vi "TestFFTOrder.vi"(8 "振动判定":T1, 9 "振动判定范围":T2, 10 "spectrum info":T3[](array[typedef]) {"x-axis units" items=["Time (s)"=0, "Frequency-CB (Hz)"=1, "Frequency-CPB (Hz)"=1248, "Frequency-Arbitrary (Hz)"=2357, "Quefrency (s)"=2, "Revolutions (rev)"=3, "Order"=4, "Speed (RPM)"=11, "Speed (rad/s)"=21, "Index"=65535]; "weighting filter" items=["Linear", "A-weighting", "B-weighting", "C-weighting", "ITU-R 468-4", "Dolby", "CCITT", "C-message", "Wb", "Wc", "Wd", "We", "Wf", "Wh", "Wj", "Wk", "Wm", "AES17 20 kHz lowpass", "AES17 40 kHz lowpass", "AES17 20 kHz highpass", "AES17 40 kHz highpass"]; "dB reference [EU]" format="%.2f"; "engineering units" items=["custom..."=0, "V"=1, "A"=21, "C"=30, "pC"=31, "s"=32, "-"=29, "Pa"=2, "N"=20, "g"=3, "m/s^2"=4, "m/s"=5, "m"=6, "mm/s"=12, "mm"=13, "micron/s"=14, "micron"=15, "in/s^2"=7, "in/s"=8, "in"=9, "mil/s"=10, "mil"=11, "rad/s^2"=16, "rad/s"=17, "rad"=18, "deg/s^2"=26, "deg/s"=27, "deg"=28, "RPM"=22, "cycle/s^2"=23, "Hz"=24, "cycle"=25, "strain"=19]; "spectral info"."window" items=["None "=0, "Hanning"=1, "Hamming"=2, "Blackman-Harris"=3, "Exact Blackman"=4, "Blackman"=5, "Flat Top"=6, "4 Term B-Harris "=7, "7 Term B-Harris"=8, "Low Sidelobe"=9, "Force - Exponential"=10, "Gaussian"=62]}, 11 "FFT 5":cluster{"x0":dbl, "dx":dbl, "Y":dbl[]}[](graph) caption="spectrum") -> (0 "Limit Specifications":cluster{"x0":dbl, "dx":dbl, "Y":dbl[]}[][](array[cluster]), 1 "数组":cluster{"freq.":dbl, "dB":dbl}[][](array[cluster]), 2 "Test Result":bool[][](array[boolean]), 3 "FFT 2":cluster{"x0":dbl, "dx":dbl, "Y":dbl[]}[](graph))   [LabVIEW 2020]
uses:
  <vilib>/measure/NI_MAPro.lvlib
  <vilib>/measure/mamon.llb/Create Continuous Mask.vi
  <vilib>/addons/_NISVFA/_Spectrum Processing/SVFA Get Spectrum Subset (1 Ch).vi
  <vilib>/addons/_NISVFA/_Spectrum Processing/SVFA Spectrum Peak Search (1 Ch).vi
  <vilib>/measure/mamon.llb/Limit Testing Frequency.vi
  <vilib>/addons/_NISVFA/_Shared subVIs/Controls/svc_Spectrum Type.ctl
  <vilib>/addons/_NISVFA/_Shared subVIs/Controls/svc_Engineering Units Text Ring.ctl
  <vilib>/addons/_NISVFA/_Shared subVIs/Controls/svc_Weighting Filter Text Ring.ctl
  <vilib>/addons/_NISVFA/_Shared subVIs/Controls/svc_X-Axis Units.ctl
  <vilib>/addons/_NISVFA/_Shared subVIs/Controls/svc_Complimentary Spectrum Units.ctl
  <vilib>/addons/_NISVFA/_Shared subVIs/Controls/svc_Spectrum Info.ctl
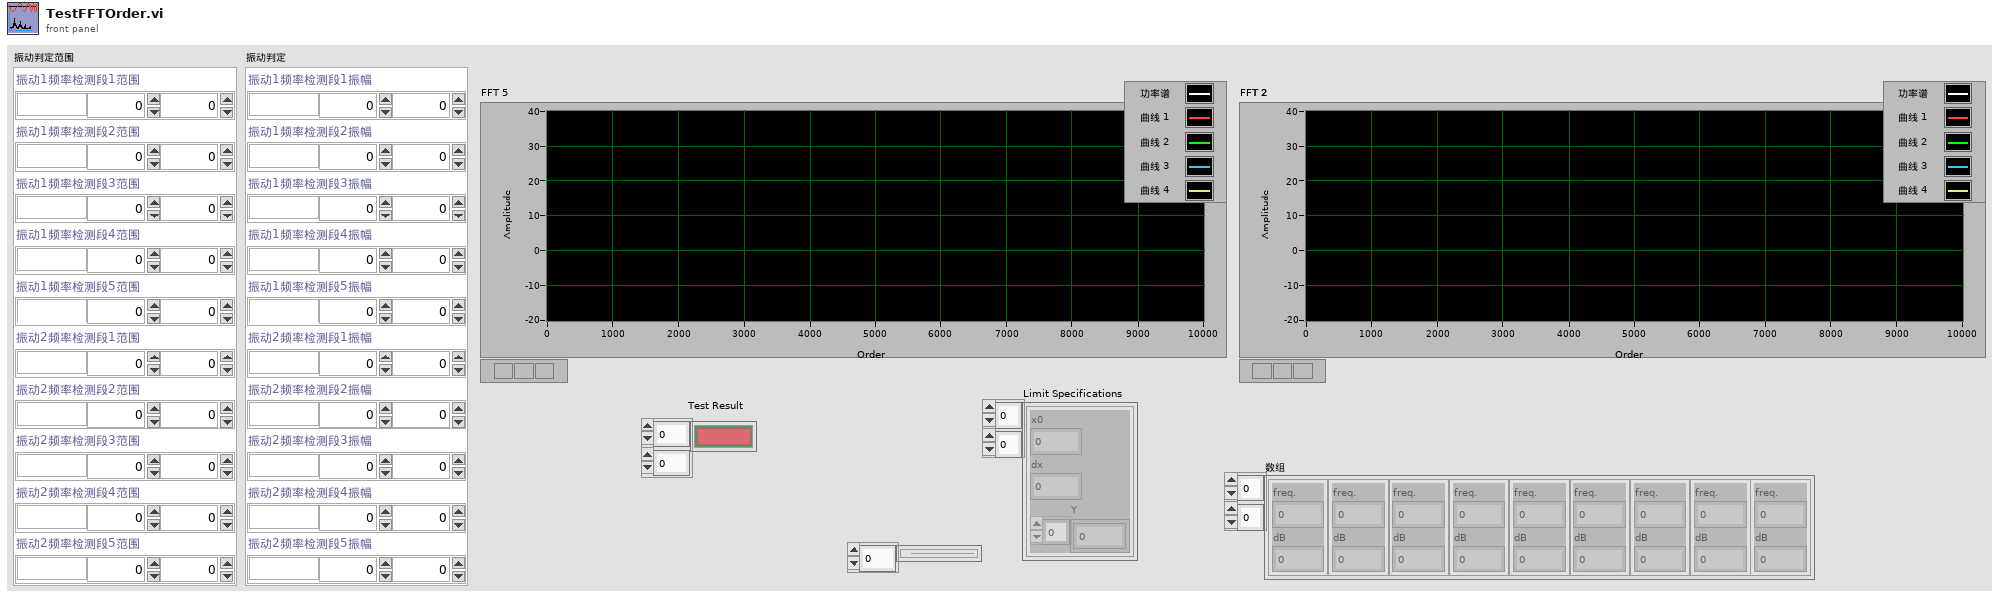
[diagram p1: front panel]
types:
  T1 = cluster{"振动1频率检测段1振幅":cluster{"单位":string, "下限":dbl, "上限":dbl}, "振动1频率检测段2振幅":cluster{"单位":string, "下限":dbl, "上限":dbl}, "振动1频率检测段3振幅":cluster{"单位":string, "下限":dbl, "上限":dbl}, "振动1频率检测段4振幅":cluster{"单位":string, "下限":dbl, "上限":dbl}, "振动1频率检测段5振幅":cluster{"单位":string, "下限":dbl, "上限":dbl}, "振动2频率检测段1振幅":cluster{"单位":string, "下限":dbl, "上限":dbl}, "振动2频率检测段2振幅":cluster{"单位":string, "下限":dbl, "上限":dbl}, "振动2频率检测段3振幅":cluster{"单位":string, "下限":dbl, "上限":dbl}, "振动2频率检测段4振幅":cluster{"单位":string, "下限":dbl, "上限":dbl}, "振动2频率检测段5振幅":cluster{"单位":string, "下限":dbl, "上限":dbl}}
  T2 = cluster{"振动1频率检测段1范围":cluster{"单位":string, "下限":dbl, "上限":dbl}, "振动1频率检测段2范围":cluster{"单位":string, "下限":dbl, "上限":dbl}, "振动1频率检测段3范围":cluster{"单位":string, "下限":dbl, "上限":dbl}, "振动1频率检测段4范围":cluster{"单位":string, "下限":dbl, "上限":dbl}, "振动1频率检测段5范围":cluster{"单位":string, "下限":dbl, "上限":dbl}, "振动2频率检测段1范围":cluster{"单位":string, "下限":dbl, "上限":dbl}, "振动2频率检测段2范围":cluster{"单位":string, "下限":dbl, "上限":dbl}, "振动2频率检测段3范围":cluster{"单位":string, "下限":dbl, "上限":dbl}, "振动2频率检测段4范围":cluster{"单位":string, "下限":dbl, "上限":dbl}, "振动2频率检测段5范围":cluster{"单位":string, "下限":dbl, "上限":dbl}}
  T3 = typedef "svc_Spectrum Info.ctl" = cluster{"channel name":string, "description":string, "x-axis units":T4, "spectral info":cluster{"spectrum type":T5, "linear/dB":enum16{"linear", "dB"}, "window":u16, "window size":i32, "FFT size":i32}, "engineering units":T6, "custom label":string, "dB reference [EU]":dbl, "peak units":enum16{"rms", "peak", "peak-peak"}, "weighting filter":T7, "spectral density?":bool, "unit label":string, "spectrum skewed?":bool, "complimentary spectrum units":T8}
  T4 = typedef "svc_X-Axis Units.ctl" = u16
  T5 = typedef "svc_Spectrum Type.ctl" = enum16{"FFT Spectrum [complex]", "Amplitude [Magnitude]", "Power [Magnitude^2]", "Cross Spectrum [complex]", "Frequency Response [Complex]"}
  T6 = typedef "svc_Engineering Units Text Ring.ctl" = u16
  T7 = typedef "svc_Weighting Filter Text Ring.ctl" = u16
  T8 = typedef "svc_Complimentary Spectrum Units.ctl" = enum16{"none", "radians", "degrees", "cycles", "imaginary"}
  T9 = cluster{"single/multiple":enum16{"Multiple Peaks", "Single Max Peak"}, "threshold":dbl}
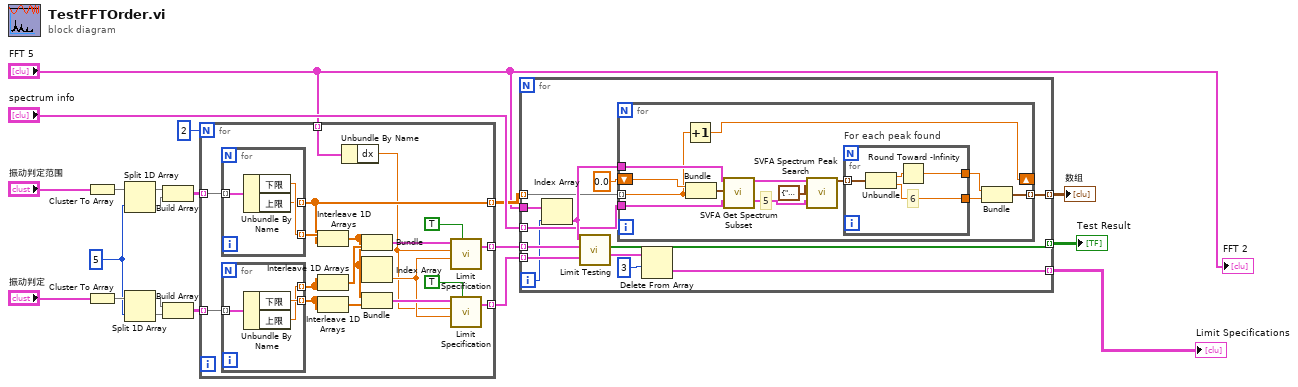
[diagram p0: block diagram]
diagram:
  w16 = 5 ("索引")
  n1 = Cluster To Array(cluster="振动判定范围") -> (array=w18:cluster{"单位":string, "下限":dbl, "上限":dbl}[])
  n2 = Cluster To Array(cluster="振动判定") -> (array=w17:cluster{"单位":string, "下限":dbl, "上限":dbl}[])
  n3 = Split 1D Array(array=w18, index=w16) -> (first subarray=w15:cluster{"单位":string, "下限":dbl, "上限":dbl}[], second subarray=w14:cluster{"单位":string, "下限":dbl, "上限":dbl}[])
  n4 = Split 1D Array(array=w17, index=w16) -> (first subarray=w13:cluster{"单位":string, "下限":dbl, "上限":dbl}[], second subarray=w12:cluster{"单位":string, "下限":dbl, "上限":dbl}[])
  n5 = Build Array(w15, w14) -> (w11:cluster{"单位":string, "下限":dbl, "上限":dbl}[][])
  n6 = Build Array(w13, w12) -> (w10:cluster{"单位":string, "下限":dbl, "上限":dbl}[][])
  n7 = for {
    N: 2 -> [_]
    tunnel: w11 -> [w37] mode=indexing
    tunnel: w10 -> [w36] mode=indexing
    tunnel: [w38] -> w5 mode=indexing
    tunnel: [w31] -> w6 mode=indexing
    tunnel: [w23] -> w4 mode=indexing
    tunnel: "FFT 5" -> [w22] mode=indexing
    n8 = for {
      tunnel: w37 -> [w44] mode=indexing
      tunnel: [w43] -> w35 mode=indexing
      tunnel: [w42] -> w23 mode=indexing
      n9 = Unbundle By Name(w44) -> ("下限"=w43:dbl, "上限"=w42:dbl)
    }
    n10 = for {
      tunnel: w36 -> [w41] mode=indexing
      tunnel: [w40] -> w34 mode=indexing
      tunnel: [w39] -> w24 mode=indexing
      n11 = Unbundle By Name(w41) -> ("下限"=w40:dbl, "上限"=w39:dbl)
    }
    n12 = Interleave 1D Arrays(w35, w23) -> (w29:dbl[])
    n13 = Interleave 1D Arrays(w24, w24) -> (w30:dbl[])
    n14 = Interleave 1D Arrays(w34, w34) -> (w28:dbl[])
    n15 = Unbundle By Name(w22) -> ("dx"=w21:dbl)
    n16 = Bundle(w29, w30) -> (w33:cluster{dbl[], dbl[]})  [unwired: 1 in]
    n17 = Index Array(array=w29) -> (element=w27:dbl)  [unwired: 1 in]
    n18 = Bundle(w29, w28) -> (w32:cluster{dbl[], dbl[]})  [unwired: 1 in]
    n19 = call-poly <vilib>:"Limit Specification.vi"("Specification Cluster"=w33, "dx"=w21, "x0"=w27, "Reset"=TRUE) -> ("Limit"=w38:cluster{"x0":dbl, "dx":dbl, "Y":dbl[]})  [unwired: 1 in, 1 out]
    n20 = call-poly <vilib>:"Limit Specification.vi"("Specification Cluster"=w32, "dx"=w21, "x0"=w27, "Reset"=TRUE) -> ("Limit"=w31:cluster{"x0":dbl, "dx":dbl, "Y":dbl[]})  [unwired: 1 in, 1 out]
  }
  n21 = for {
    tunnel: [w55] -> w9 mode=indexing
    tunnel: [w47] -> w8 mode=indexing
    tunnel: "FFT 5" -> [w54]
    tunnel: "spectrum info" -> [w53] mode=indexing
    tunnel: w6 -> [w46] mode=indexing
    tunnel: w5 -> [w52] mode=indexing
    tunnel: w4 -> [w51] mode=indexing
    tunnel: [w48] -> w1 mode=indexing
    i -> [w45]
    n22 = Index Array(array=w54, index=w45) -> (element=w57:cluster{"x0":dbl, "dx":dbl, "Y":dbl[]})
    n23 = call-poly <vilib>:"Limit Testing.vi"("lower limit"=w46, "upper limit"=w52, "signal in"=w57) -> ("output values"=w50:cluster{"x0":dbl, "dx":dbl, "Y":dbl[]}[], "test results"=w47:bool[])  [unwired: 3 in, 4 out]
    n24 = for {
      tunnel: w57 -> [w70]
      tunnel: w53 -> [w69]
      tunnel: w51 -> [w60] mode=indexing
      shift-right: [w59] -> _
      shift-left: 0.0 -> [w64]
      tunnel: [w63] -> w55 mode=indexing
      # "5"
      n25 = Increment(x=w60) -> (x+1=w59:dbl)
      n26 = Bundle(w64, "上限"=w60) -> (w68:cluster{dbl, "上限":dbl})  [unwired: 1 in]
      n27 = call-poly <vilib>:"SVFA Get Spectrum Subset.vi"("spectrum"=w70, "range"=w68, "spectrum info"=w69) -> ("spectrum subset"=w58:cluster{"x0":dbl, "dx":dbl, "magnitude":dbl[]}, "dup spectrum info"=w62:T3)  [unwired: 11 in, 4 out]
      n28 = call-poly <vilib>:"SVFA Spectrum Peak Search.vi"("spectrum"=w58, "peak search settings"=T9 {"single/multiple"=enum."Single Max Peak", "threshold"=0.0}, "spectrum info in"=w62) -> ("peaks"=w66:cluster{"freq. or order":dbl, "value":dbl}[])  [unwired: 12 in, 4 out]
      n29 = for "For each peak found" {
        tunnel: w66 -> [w74] mode=indexing
        tunnel: [w72] -> w65
        tunnel: [w73] -> w61
        # "6"
        n30 = Unbundle(w74) -> ("freq. or order"=w71:dbl, "value"=w73:dbl)
        n31 = Round Toward -Infinity(1:w71) -> (0:w72:dbl)
      }
      n32 = Bundle(w65, "value"=w61) -> (w63:cluster{dbl, "value":dbl})  [unwired: 1 in]
    }
    n33 = Delete From Array(array=w50, length=3 ("长度")) -> (deleted portion=w48:cluster{"x0":dbl, "dx":dbl, "Y":dbl[]}[])  [unwired: 1 in, 1 out]
  }
  "数组" <- w9
  "Test Result" <- w8
  "Limit Specifications" <- w1
  "FFT 2" <- "FFT 5"
